vi "_RunCalMethod.vi"(4 "Method":T1={"Lenses"=[{"Scan Type"=0, "Scans"=1000, "Time 1"=0.0, "Time 2"=5.0, "Value 1"=400.0, "Value 2"=400.0, "Step Size"=1.0}, {"Scan Type"=0, "Scans"=1, "Time 1"=1.0, "Time 2"=1.0, "Value 1"=600.0, "Value 2"=600.0, "Step Size"=1.0}, {"Scan Type"=0, "Scans"=1, "Time 1"=1.0, "Time 2"=1.0, "Value 1"=32000.0, "Value 2"=32000.0, "Step Size"=1.0}, {"Scan Type"=0, "Scans"=1, "Time 1"=1.0, "Time 2"=1.0, "Value 1"=400.0, "Value 2"=400.0, "Step Size"=1.0}, {"Scan Type"=0, "Scans"=1, "Time 1"=1.0, "Time 2"=1.0, "Value 1"=600.0, "Value 2"=600.0, "Step Size"=1.0}, {"Scan Type"=0, "Scans"=1, "Time 1"=1.0, "Time 2"=1.0, "Value 1"=32000.0, "Value 2"=32000.0, "Step Size"=1.0}, {"Scan Type"=0, "Scans"=1, "Time 1"=1.0, "Time 2"=1.0, "Value 1"=500.0, "Value 2"=400.0, "Step Size"=1.0}, {"Scan Type"=0, "Scans"=1, "Time 1"=1.0, "Time 2"=1.0, "Value 1"=70.0, "Value 2"=80.0, "Step Size"=1.0}, {"Scan Type"=0, "Scans"=1, "Time 1"=1.0, "Time 2"=1.0, "Value 1"=80.0, "Value 2"=80.0, "Step Size"=1.0}, {"Scan Type"=0, "Scans"=1, "Time 1"=1.0, "Time 2"=1.0, "Value 1"=-1.0, "Value 2"=100.0, "Step Size"=1.0}, {"Scan Type"=0, "Scans"=1, "Time 1"=1.0, "Time 2"=1.0, "Value 1"=-2.0, "Value 2"=100.0, "Step Size"=1.0}, {"Scan Type"=0, "Scans"=1, "Time 1"=1.0, "Time 2"=1.0, "Value 1"=-3.0, "Value 2"=100.0, "Step Size"=1.0}, {"Scan Type"=0, "Scans"=1, "Time 1"=1.0, "Time 2"=1.0, "Value 1"=-4.0, "Value 2"=100.0, "Step Size"=1.0}, {"Scan Type"=0, "Scans"=1, "Time 1"=1.0, "Time 2"=1.0, "Value 1"=-15.0, "Value 2"=100.0, "Step Size"=1.0}, {"Scan Type"=0, "Scans"=1, "Time 1"=1.0, "Time 2"=1.0, "Value 1"=-4.5, "Value 2"=-9.0, "Step Size"=1.0}, {"Scan Type"=0, "Scans"=1, "Time 1"=1.0, "Time 2"=1.0, "Value 1"=0.0, "Value 2"=100.0, "Step Size"=1.0}, {"Scan Type"=0, "Scans"=1, "Time 1"=1.0, "Time 2"=1.0, "Value 1"=-100.0, "Value 2"=100.0, "Step Size"=1.0}, {"Scan Type"=0, "Scans"=1, "Time 1"=1.0, "Time 2"=1.0, "Value 1"=-50.0, "Value 2"=100.0, "Step Size"=1.0}, {"Scan Type"=0, "Scans"=1, "Time 1"=1.0, "Time 2"=1.0, "Value 1"=100.0, "Value 2"=100.0, "Step Size"=1.0}, {"Scan Type"=0, "Scans"=1, "Time 1"=1.0, "Time 2"=1.0, "Value 1"=-51.0, "Value 2"=100.0, "Step Size"=1.0}, {"Scan Type"=0, "Scans"=1, "Time 1"=1.0, "Time 2"=1.0, "Value 1"=-62.0, "Value 2"=100.0, "Step Size"=1.0}, {"Scan Type"=0, "Scans"=1, "Time 1"=1.0, "Time 2"=1.0, "Value 1"=-52.0, "Value 2"=-150.0, "Step Size"=1.0}, {"Scan Type"=0, "Scans"=1, "Time 1"=1.0, "Time 2"=1.0, "Value 1"=-100.0, "Value 2"=-200.0, "Step Size"=1.0}, {"Scan Type"=0, "Scans"=1, "Time 1"=1.0, "Time 2"=1.0, "Value 1"=15.0, "Value 2"=50.0, "Step Size"=1.0}, {"Scan Type"=0, "Scans"=1, "Time 1"=1.0, "Time 2"=1.0, "Value 1"=2000.0, "Value 2"=500.0, "Step Size"=1.0}, {"Scan Type"=0, "Scans"=1, "Time 1"=1.0, "Time 2"=1.0, "Value 1"=5500.0, "Value 2"=1000.0, "Step Size"=1.0}, {"Scan Type"=0, "Scans"=1, "Time 1"=1.0, "Time 2"=1.0, "Value 1"=420.0, "Value 2"=420.0, "Step Size"=1.0}, {"Scan Type"=0, "Scans"=1, "Time 1"=1.0, "Time 2"=1.0, "Value 1"=-420.0, "Value 2"=-420.0, "Step Size"=1.0}, {"Scan Type"=0, "Scans"=1, "Time 1"=1.0, "Time 2"=1.0, "Value 1"=420.0, "Value 2"=420.0, "Step Size"=1.0}, {"Scan Type"=0, "Scans"=1, "Time 1"=1.0, "Time 2"=1.0, "Value 1"=-420.0, "Value 2"=-420.0, "Step Size"=1.0}, {"Scan Type"=0, "Scans"=1, "Time 1"=1.0, "Time 2"=1.0, "Value 1"=600.0, "Value 2"=600.0, "Step Size"=1.0}, {"Scan Type"=0, "Scans"=1, "Time 1"=1.0, "Time 2"=1.0, "Value 1"=-600.0, "Value 2"=600.0, "Step Size"=1.0}, {"Scan Type"=0, "Scans"=1, "Time 1"=1.0, "Time 2"=1.0, "Value 1"=80.0, "Value 2"=0.9, "Step Size"=1.0}, {"Scan Type"=0, "Scans"=1, "Time 1"=1.0, "Time 2"=1.0, "Value 1"=90.0, "Value 2"=0.0, "Step Size"=1.0}, {"Scan Type"=0, "Scans"=1, "Time 1"=1.0, "Time 2"=1.0, "Value 1"=0.0, "Value 2"=0.0, "Step Size"=1.0}, {"Scan Type"=0, "Scans"=1, "Time 1"=1.0, "Time 2"=1.0, "Value 1"=0.0, "Value 2"=0.0, "Step Size"=1.0}, {"Scan Type"=0, "Scans"=1, "Time 1"=1.0, "Time 2"=1.0, "Value 1"=0.0, "Value 2"=0.0, "Step Size"=1.0}, {"Scan Type"=0, "Scans"=1, "Time 1"=1.0, "Time 2"=1.0, "Value 1"=0.0, "Value 2"=0.0, "Step Size"=1.0}, {"Scan Type"=0, "Scans"=1, "Time 1"=1.0, "Time 2"=1.0, "Value 1"=500.0, "Value 2"=0.0, "Step Size"=1.0}, {"Scan Type"=0, "Scans"=1, "Time 1"=1.0, "Time 2"=1.0, "Value 1"=0.0, "Value 2"=0.0, "Step Size"=1.0}, {"Scan Type"=0, "Scans"=1, "Time 1"=1.0, "Time 2"=1.0, "Value 1"=5850.0, "Value 2"=0.0, "Step Size"=1.0}, {"Scan Type"=0, "Scans"=1, "Time 1"=1.0, "Time 2"=1.0, "Value 1"=0.0, "Value 2"=0.0, "Step Size"=1.0}, {"Scan Type"=0, "Scans"=1, "Time 1"=1.0, "Time 2"=1.0, "Value 1"=1000.0, "Value 2"=0.0, "Step Size"=1.0}, {"Scan Type"=0, "Scans"=1, "Time 1"=1.0, "Time 2"=1.0, "Value 1"=320.0, "Value 2"=0.0, "Step Size"=1.0}, {"Scan Type"=0, "Scans"=1, "Time 1"=1.0, "Time 2"=1.0, "Value 1"=0.0, "Value 2"=0.0, "Step Size"=1.0}, {"Scan Type"=0, "Scans"=1, "Time 1"=1.0, "Time 2"=1.0, "Value 1"=0.0, "Value 2"=0.0, "Step Size"=1.0}], "Mass Ranges"=[{"Start"=54.0, "Stop"=64.0, "Step Size"=0.1, "Steps"=101, "Dwell"=10.0, "Parameters"=[], "Res"=1}, {"Start"=170.0, "Stop"=180.0, "Step Size"=0.1, "Steps"=101, "Dwell"=10.0, "Parameters"=[], "Res"=1}, {"Start"=611.0, "Stop"=621.0, "Step Size"=0.1, "Steps"=101, "Dwell"=10.0, "Parameters"=[], "Res"=1}, {"Start"=902.0, "Stop"=912.0, "Step Size"=0.1, "Steps"=101, "Dwell"=10.0, "Parameters"=[], "Res"=1}, {"Start"=1250.0, "Stop"=1260.0, "Step Size"=0.1, "Steps"=101, "Dwell"=10.0, "Parameters"=[], "Res"=1}, {"Start"=1540.0, "Stop"=1550.0, "Step Size"=0.1, "Steps"=101, "Dwell"=10.0, "Parameters"=[], "Res"=1}, {"Start"=1773.0, "Stop"=1783.0, "Step Size"=0.1, "Steps"=101, "Dwell"=10.0, "Parameters"=[], "Res"=1}, {"Start"=2005.0, "Stop"=2015.0, "Step Size"=0.1, "Steps"=101, "Dwell"=10.0, "Parameters"=[], "Res"=1}], "Acquire"=FALSE, "MCA"=FALSE, "Q1DC EN"=FALSE, "Q1 POL"=FALSE, "Q3 POL"=FALSE, "Q1 RF  EN"=TRUE, "Averaging"=FALSE, "Log Scale"=FALSE, "CPS"=TRUE, "Unit"=FALSE, "Data Path"=path "", "Run Mode"=enum."Q1 Scan", "Fixed Mass (amu)"=609.2, "Q3DC EN"=FALSE, "Q3 RF  EN"=TRUE, "Negative"=FALSE} {"Mass Ranges"."Res" items=["High/High", "Medium/Medium", "Low/Low", "High/Medium", "High/Low", "Medium/High", "Medium/Low", "Low/High", "Low/Medium"]}, 6 "millisecond timer value":u32, 7 "Pause":refnum<vi>) -> (0 "error out":errorcluster)   [LabVIEW 2015]
uses:
  Type/_GUI Method.ctl
  Type/_Lens Property.ctl
  Type/_Mass Range Property.ctl
  Type/_Mass Range Parameters.ctl
  Type/_RT Res Type.ctl
  Type/_Run Mode.ctl
  Type/_Run Module.ctl
  Configuration/_Global Configuration.vi
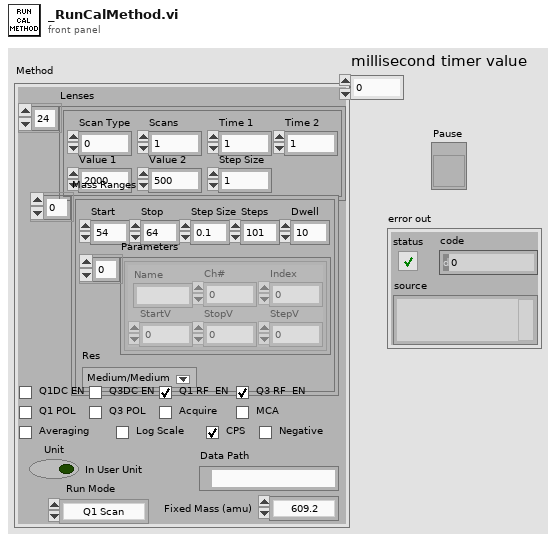
[diagram p1: front panel]
types:
  T1 = typedef "_GUI Method.ctl" = cluster{"Lenses":T2[], "Mass Ranges":T3[], "Acquire":bool, "MCA":bool, "Q1DC EN":bool, "Q1 POL":bool, "Q3 POL":bool, "Q1 RF  EN":bool, "Averaging":bool, "Log Scale":bool, "CPS":bool, "Unit":bool, "Data Path":path, "Run Mode":T6, "Fixed Mass (amu)":dbl, "Q3DC EN":bool, "Q3 RF  EN":bool, "Negative":bool}
  T2 = typedef "_Lens Property.ctl" = cluster{"Scan Type":u8, "Scans":i32, "Time 1":dbl, "Time 2":dbl, "Value 1":dbl, "Value 2":dbl, "Step Size":dbl}
  T3 = typedef "_Mass Range Property.ctl" = cluster{"Start":dbl, "Stop":dbl, "Step Size":dbl, "Steps":i32, "Dwell":dbl, "Parameters":T4[], "Res":T5}
  T4 = typedef "_Mass Range Parameters.ctl" = cluster{"Name":string, "Ch#":u8, "StartV":dbl, "StopV":dbl, "StepV":dbl, "Index":u8}
  T5 = typedef "_RT Res Type.ctl" = u16
  T6 = typedef "_Run Mode.ctl" = enum16{"MRM (Q1/Q2)", "Q1 Scan", "Q1 SRM", "Q2 Scan", "Q2 SRM", "Product Scan", "Precursor Scan", "Neutral Loss", "Neutral Gain"}
  T7 = enum32{"Bad", "Idle", "Run top level", "Running"}
  T8 = typedef "_Run Module.ctl" = u16
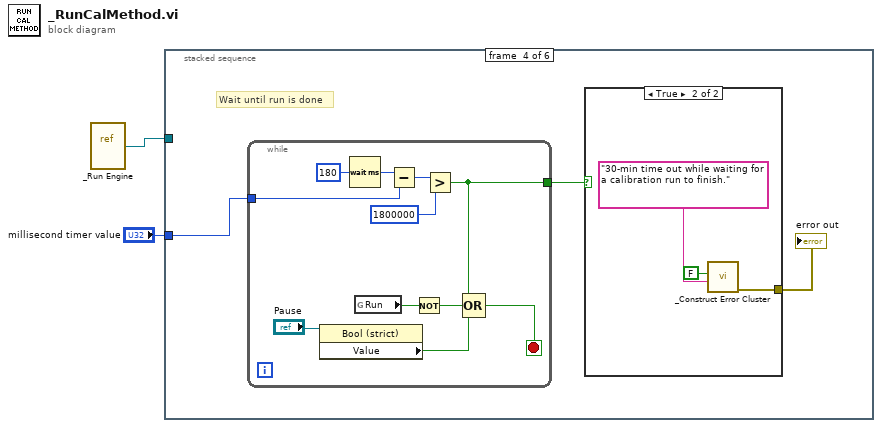
[diagram p0: block diagram]
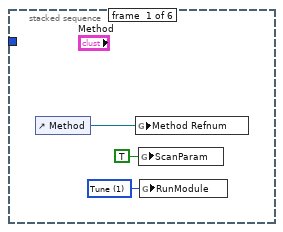
[diagram p2: hidden frame]
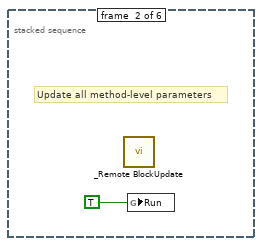
[diagram p3: hidden frame]
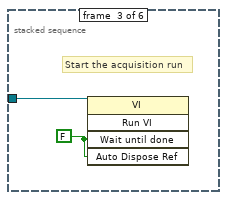
[diagram p4: hidden frame]
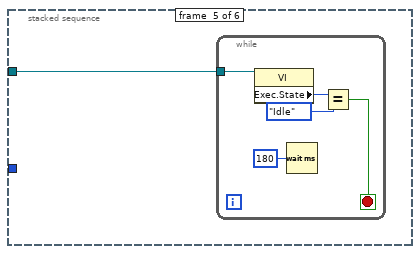
[diagram p6: hidden frame]
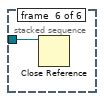
[diagram p7: hidden frame]
diagram:
  n1 = vi-ref "_Run Engine.vi"() -> (w2:refnum<vi>)
  n2 = stacked-sequence {
    tunnel: w2 -> [_ _ w7 _ w26 w32]
    tunnel: "millisecond timer value" -> [_ _ _ w9 _ _]
    frame #0 {
      w4 = T8 1 items=["Diagnostics", "Tune", "Acquisition"] ("RunModule")
      n3 = control-ref of="Method"() -> (w3:refnum<vi>)
      n4 = global write "_Global Configuration.vi" "Method Refnum"(w3) -> ()
      n5 = global write "_Global Configuration.vi" "ScanParam"(TRUE ("ScanParam")) -> ()
      n6 = global write "_Global Configuration.vi" "RunModule"(w4) -> ()
    }
    frame #1 {
      # "Update all method-level parameters"
      n7 = call "_Remote BlockUpdate.vi"() -> ()  [unwired: 3 in, 5 out]
      n8 = global write "_Global Configuration.vi" "Run"(TRUE ("Update")) -> ()
    }
    frame #2 {
      w8 = FALSE ("Wait until done")
      # "Start the acquisition run"
      n9 = invoke class="VI" method="Run VI"(reference=w7, "Wait until done"=w8, "Auto Dispose Ref"=w8) -> ()  [unwired: 2 in, 5 out]
    }
    frame #3 {
      # "Wait until run is done"
      n10 = while {
        tunnel: w9 -> [w23]
        tunnel: [w17] -> w11
        stop <- w19 stop-if-true
        n11 = property class="Bool (strict)"(reference="Pause") -> ("Value"=w15:bool)  [unwired: 1 in, 2 out]
        n12 = Wait (ms)(milliseconds to wait=u32 180) -> (millisecond timer value=w24:u32)
        n13 = global read "_Global Configuration.vi" "Run"() -> (w20:bool)
        n14 = Subtract(x=w24, y=w23) -> (x-y=w22:u32)
        n15 = Not(x=w20) -> (.not. x?=w18:bool)
        n16 = Greater?(x=w22, y=u32 1800000) -> (0:w17:bool)
        n17 = Compound Arithmetic op=OR(w17, w18, w15) -> (w19:bool)
      }
      n18 = case shown="True" w11 {
        tunnel: [_ w13] -> w10
        frame False {
        }
        frame True {
          n19 = call "_Construct Error Cluster.vi"("reason"="30-min time out while waiting for a calibration run to finish.", "CallingChain? (T)"=FALSE) -> ("error out"=w13:errorcluster)  [unwired: 5 in]
        }
      }
      "error out" <- w10
    }
    frame #4 {
      n20 = while {
        tunnel: w26 -> [w31]
        stop <- w28 stop-if-true
        n21 = property class="VI"(reference=w31) -> ("Exec.State"=w30:T7)  [unwired: 1 in, 2 out]
        n22 = Wait (ms)(milliseconds to wait=u32 180) -> ()  [unwired: 1 out]
        n23 = Equal?(x=w30, y=T7."Idle") -> (x = y?=w28:bool)
      }
    }
    frame #5 {
      n24 = Close Reference(reference=w32) -> ()  [unwired: 1 in, 1 out]
    }
  }
